vi "StartSlideOut.vi"(8 "error in (no error)":errorcluster, 10 "Engine in":refnum<class "Engine.lvclass">, 11 "Menu in":refnum<class "Menu.lvclass">) -> (0 "error out":errorcluster, 2 "Engine out":refnum<class "Engine.lvclass">, 3 "Menu out":refnum<class "Menu.lvclass">)   [LabVIEW 2019, in "RT_Game.lvlib" / "Menu.lvclass"]
uses:
  Menu.lvclass
  C:/Users/FreshBob/Dropbox/VIs/myRIO_GameConsole/RT/RT_Game/Game/Game.lvclass
  Engine/Engine.lvclass
  States.ctl
  Menu.lvclass/Menu.ctl
  Game/Game.lvclass/Game.ctl
  Game/Write State.vi
  Game/Game.lvclass
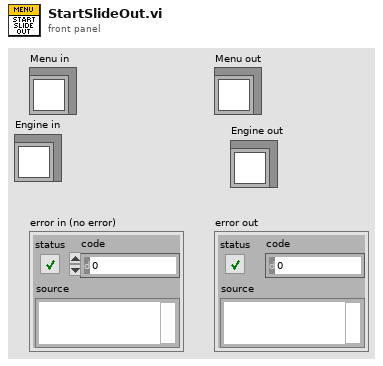
[diagram p1: front panel]
types:
  T1 = typedef "RT_Game.lvlib/Game.lvclass/States.ctl" = enum16{"Init", "Restart", "Menu", "Game", "Resume", "ToggleSingleplayer", "LoadNextGame", "ExitToMenu", "NewHighscore", "GameOver", "SlideOut"}
  T2 = typedef "RT_Game.lvlib/Game.lvclass/ScreenSide.ctl" = enum16{"up", "down", "left", "right", "none"}
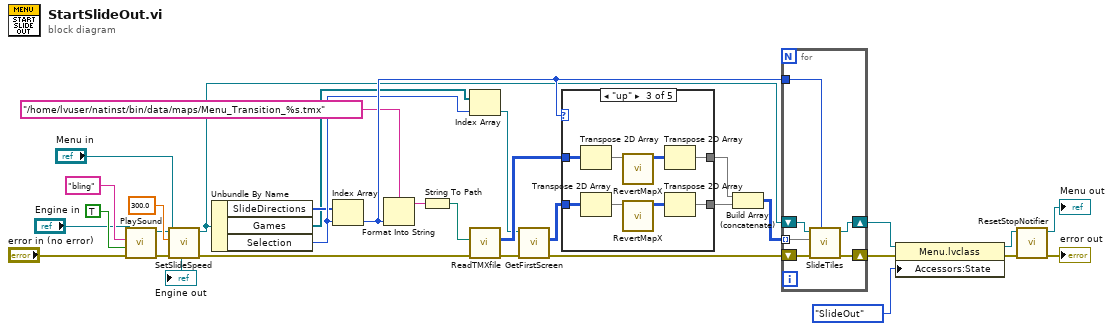
[diagram p0: block diagram]
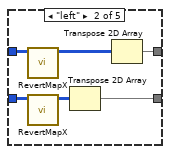
[diagram p3: hidden frame]
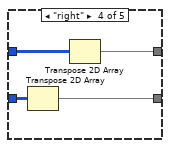
[diagram p4: hidden frame]
diagram:
  n1 = call "PlaySound.vi"("error in (no error)"="error in (no error)", "Overwrite"=TRUE, "Name"="bling", "Engine in"="Engine in") -> ("error out"=w9:errorcluster, "Engine out"=→"Engine out":refnum<class "Engine.lvclass">)  [unwired: 6 in]
  n2 = call "SetSlideSpeed.vi"("error in (no error)"=w9, "Speed_x"=300.0, "Game in"="Menu in") -> ("error out"=w15:errorcluster, "Game out"=w16:refnum<class "Menu.lvclass">)  [unwired: 7 in]
  n3 = Unbundle By Name(w16) -> ("SlideDirections"=w23:T2[], "Games"=w12:refnum<class "Game.lvclass">[], "Selection"=w24:i8)
  n4 = Index Array(array=w23, index=w24) -> (element=w29:T2)
  n5 = Format Into String(format string="/home/lvuser/natinst/bin/data/maps/Menu_Transition_%s.tmx", w29) -> (resulting string=w26:string)  [unwired: 2 in, 1 out]
  n6 = String To Path(string=w26) -> (path=w27:path)
  n7 = Index Array(array=w12, index=w24) -> (element=w14:refnum<class "Game.lvclass">)
  n8 = call "ReadTMXfile.vi"("error in (no error)"=w15, "path to tmx-file (created with Tiles2D)"=w27) -> ("error out"=w10:errorcluster, "Tilenumbers"=w28:u32[][])  [unwired: 8 in]
  n9 = call-dynamic "GetFirstScreen.vi"("error in (no error)"=w10, "Game in"=w14) -> ("error out"=w13:errorcluster, "Array"=w30:u32[][])  [unwired: 7 in, 1 out]
  n10 = case shown="\"up\"" w29 {
    tunnel: w28 -> [w34 w40 w42 w52 w54]
    tunnel: [w34 w36 w41 w50 w54] -> w31
    tunnel: w30 -> [w33 w38 w48 w51 w53]
    tunnel: [w33 w35 w45 w49 w53] -> w32
    frame Default {
    }
    frame "left" {
      n11 = call "RevertMapX.vi"("Tilenumbers"=w40) -> ("Array"=w39:u32[][])  [unwired: 10 in]
      n12 = call "RevertMapX.vi"("Tilenumbers"=w38) -> ("Array"=w37:u32[][])  [unwired: 10 in]
      n13 = Transpose 2D Array(2D array=w37) -> (transposed array=w35:u32[][])
      n14 = Transpose 2D Array(2D array=w39) -> (transposed array=w36:u32[][])
    }
    frame "up" {
      n15 = Transpose 2D Array(2D array=w42) -> (transposed array=w44:u32[][])
      n16 = Transpose 2D Array(2D array=w48) -> (transposed array=w46:u32[][])
      n17 = call "RevertMapX.vi"("Tilenumbers"=w44) -> ("Array"=w43:u32[][])  [unwired: 10 in]
      n18 = call "RevertMapX.vi"("Tilenumbers"=w46) -> ("Array"=w47:u32[][])  [unwired: 10 in]
      n19 = Transpose 2D Array(2D array=w43) -> (transposed array=w41:u32[][])
      n20 = Transpose 2D Array(2D array=w47) -> (transposed array=w45:u32[][])
    }
    frame "right" {
      n21 = Transpose 2D Array(2D array=w51) -> (transposed array=w49:u32[][])
      n22 = Transpose 2D Array(2D array=w52) -> (transposed array=w50:u32[][])
    }
    frame "down" {
    }
  }
  n23 = Build Array (concatenate)(w31, w32) -> (w18:u32[][])
  n24 = for {
    shift-right: [w59] -> w11
    shift-left: w13 -> [w60]
    shift-right: [w58] -> w20
    shift-left: w16 -> [w57]
    tunnel: w29 -> [w56]
    tunnel: w18 -> [w55] mode=indexing
    n25 = call "SlideTiles.vi"("Side"=w56, "error in (no error)"=w60, "Tilecodes"=w55, "Game in"=w57) -> ("error out"=w59:errorcluster, "Game out"=w58:refnum<class "Menu.lvclass">)  [unwired: 6 in]
  }
  n26 = property class="Menu.lvclass"(reference=w20, error in=w11, "Accessors:State"=States."SlideOut" ("State")) -> (reference out=w22:refnum<class "Menu.lvclass">, error out=w19:errorcluster)
  n27 = call "ResetStopNotifier.vi"("error in (no error)"=w19, "Game in"=w22) -> ("error out"=→"error out":errorcluster, "Game out"=→"Menu out":refnum<class "Menu.lvclass">)  [unwired: 8 in]
